vi "Reset Measurement List Display.vi"(8 "error in (no error)":errorcluster, 11 "Server UI in":refnum<class "Server UI.lvclass">) -> (0 "error out":errorcluster, 3 "Server UI out":refnum<class "Server UI.lvclass">)   [LabVIEW 2026, in "Server UI.lvlib" / "Server UI.lvclass"]
uses:
  Server UI.lvclass
  C:/Users/E2013170/Documents/GitHub/Measurement-Utility-Reference/source/framework/Msmt UI/Measurement UI.lvclass
  framework/Msmt UI/Measurement UI.lvclass/Measurement UI.ctl
  framework/Msmt UI/Accessors/Read Measurement.vi
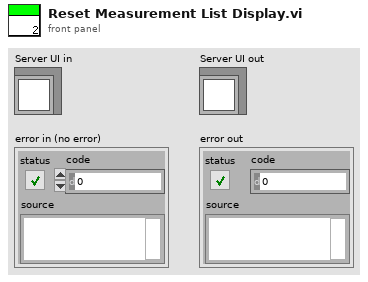
[diagram p1: front panel]
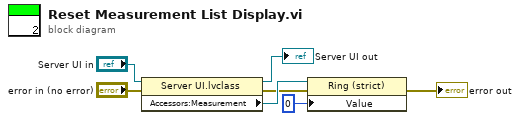
[diagram p0: block diagram]
diagram:
  n1 = property on="Property Node" class="Server UI.lvclass"(reference="Server UI in", error in="error in (no error)") -> (reference out=→"Server UI out":refnum<class "Server UI.lvclass">, error out=w2:errorcluster, "Accessors:Measurement"=w5:refnum<vi>)
  n2 = property on="Property Node" class="Ring (strict)"(reference=w5, error in=w2, "Value"=u16 0) -> (error out=→"error out":errorcluster)  [unwired: 1 out]
